vi "240312_frequency_sweep.vi"() -> ()   [LabVIEW 2015]
uses:
  <vilib>/Utility/error.llb/DialogTypeEnum.ctl
  Libraries/Stanford Research SG39x Series/Stanford Research SG39x Series.lvlib
  Libraries/SR400/SR400.lvlib
  Libraries/SRS_SR400(2013)/SRS SR400.lvlib
panel:
  out "1 cycle done":bool
  out "measure done":bool
  in  "start measurement":bool caption="Start measure"
  out "How to make setting default":string="우클릭 -> Data Operations -> Make Current Value Default"
  in  "Control":T1(tab)
  out "Parameter Explanation":string="Number of samples : 몇 번 accumulate 할 것인가에 대한 값, T SET에 해당한다.\nGate X width/delay : trigger 이후에 언제의 값을 측정할 것인가에 해당한다.\n\n>>이외에 설정값은 sub vi에서 자동으로 설정된다. 만일 바꾸고 싶다면, 해당 값을 설정하라. 세팅하면서 겪은 시행착오에 대해 sub-vi에서 건드는 값에 대해 간략히 설명해두도록 하겠다.\n>> 아래로 쭉 내용 있음\n>> 혹시라도 트리거가 제대로 들어가지 않는다면, Window->Show block diagram에서 SR400의 trigger level을 좀 낮춰보도록 하라. 거의 그럴 일은 없을 것이다.. 다만, 이 경우는 AFG를 통해 컨트롤을 한다면 참고하는 것이 좋을 것이다. \n>> Set Disc level : 이 값은 기본적으로 0.3V로 설정된다. 너무 작으면 제대로 count를 하지 못한다.\n>> Dwell time : SR400의 N_period 값이 1이 아닌 경우, 다음 스텝이 시작될 때 까지 얼마나 기다릴 것인가와 관련된다. \n                      우리의 세팅에서는 큰 의미가 없다. 한 번 trigger가 올라갔을 때 얼마나 카운팅 할 것인가에 대한 값이다.\n                      궁금하다면 바탕화면의 매뉴얼을 참고하라.\n>> N period : T_set만큼 accumulate 하는 것을 몇 번 할 것인가에 대한 값이다. 우리는 그닥 신경 안써도 된다. \n>> Gate mode : Fixed가 기본이다. 지정된 delay부터 width만큼만 값을 읽겠다는 것이다. CW는 그냥 trigger가 들어오는 시간동안 쭉 재겠다는\n                      것이다.\n>> Counter Presets : T로 되어있는데, T값을 통해 트리거하겠다는 느낌으로 생각하면 된다. 이 값은 건들 일 없을 것이다. 더 자세하게 궁금하면\n                             장비 매뉴얼을 참고하라.\n>> 나머지 값들은 장비 매뉴얼을 보거나 직접 건드려보는 편이 훨씬 더 간편하게 습득할 수 있다. \n>> EOF"
  out "String 2":string="Initialize"
  in  "SR_400_GPIB_ADDR":refnum<visa-resource-name>="GPIB0::18::INSTR"
  in  "Number of samples":dbl=5000.0
  in  "Gate B width":dbl[unit]=3e-05
  in  "Gate A width":dbl[unit]=3e-05
  in  "Gate B delay":dbl[unit]=6.03e-05
  in  "Gate A delay":dbl[unit]=3.0000000000000004e-07
  out "String":string="Measurement Setting"
  out "String 3":string="Initialize"
  in  "Final frequency (<3940MHz)":dbl=3500.0
  in  "Frequency step (MHz)":dbl=100.0
  in  "Initial frequency (<3940MHz)":dbl=2500.0 format="%#_13g"
  in  "SG394_GPIB_ADDR":refnum<visa-resource-name>="GPIB0::20::INSTR"
  in  "Modulation type":u16(ring)=7 items=["AM/ASK"=0, "FM/FSK"=1, "PM/PSK"=2, "Sweep"=3, "Pulse"=4, "Blank"=5, "QAM"=7, "CPM"=8, "VSB"=9]
  in  "N type output level value (-136dBm to 0 dBm)":dbl
  in  "start PB":bool
  in  "stop PB":bool
  in  "clock_freq (MHz)":dbl=500.0
  in  "# of Instructions":u32=4
  in  "Path to spinapi.dll":path=path "C:/SpinCore/SpinAPI/dll/spinapi64.dll"
  in  "Instructions":T2(array[cluster])=[{"Instruct Data"=0, "Op Code"=0, "Flags"=[TRUE, FALSE, FALSE, FALSE, FALSE, FALSE, FALSE, FALSE, FALSE, FALSE, FALSE, FALSE, FALSE, FALSE, FALSE, FALSE, FALSE, FALSE, FALSE, FALSE, FALSE, FALSE, FALSE, FALSE], "Comments"="", "Time (s)"=0.1}, {"Instruct Data"=0, "Op Code"=0, "Flags"=[FALSE, FALSE, FALSE, FALSE, FALSE, FALSE, FALSE, FALSE, FALSE, FALSE, FALSE, FALSE, FALSE, FALSE, FALSE, FALSE, FALSE, FALSE, FALSE, FALSE, FALSE, FALSE, FALSE, FALSE], "Comments"="", "Time (s)"=0.1}, {"Instruct Data"=0, "Op Code"=0, "Flags"=[TRUE, FALSE, FALSE, FALSE, FALSE, FALSE, FALSE, FALSE, FALSE, FALSE, FALSE, FALSE, FALSE, FALSE, FALSE, FALSE, FALSE, FALSE, FALSE, FALSE, FALSE, FALSE, FALSE, FALSE], "Comments"="", "Time (s)"=0.1}, {"Instruct Data"=0, "Op Code"=6, "Flags"=[FALSE, FALSE, FALSE, FALSE, FALSE, FALSE, FALSE, FALSE, FALSE, FALSE, FALSE, FALSE, FALSE, FALSE, FALSE, FALSE, FALSE, FALSE, FALSE, FALSE, FALSE, FALSE, FALSE, FALSE], "Comments"="", "Time (s)"=0.1}] {"Time (s)" format="%.3p"; "Op Code" items=["Continue", "Stop", "Loop", "End Loop", "JSR", "RTS", "Branch", "Long Delay", "Wait"]}
  in  "load":bool
  in  "board_num":i32
  in  "change board":bool
  out "Current frequency (MHz)":dbl
  out "Count A":i32
  out "Count B":i32
  in  "file path for measurement parameters":path=path "C:/Users/Choi group/Dropbox/Labbook/Quantum Optics/hBN/230726/attoDRY/parameters log.txt"
  in  "Parameters logging?\nMake block diagram if you want":bool=TRUE
  out "output file":refnum<file>
  in  "Measurement #":i32=11
  in  "No File Out?":bool
  in  "file folder path":path=path "C:/Users/resolution/Desktop/NV_measurements/test"
  # "1"
  # "2"
  # "3"
  # "4"
  # "5"
  # "6"
  # "7"
  # "8"
  # "9"
  # "10"
  # "11"
  # "12"
  # "13"
  # "14"
  # "15"
  # "16"
  # "17"
  # "18"
  # "19"
  # "20"
  # "21"
  # "22"
  # "23"
  # "24"
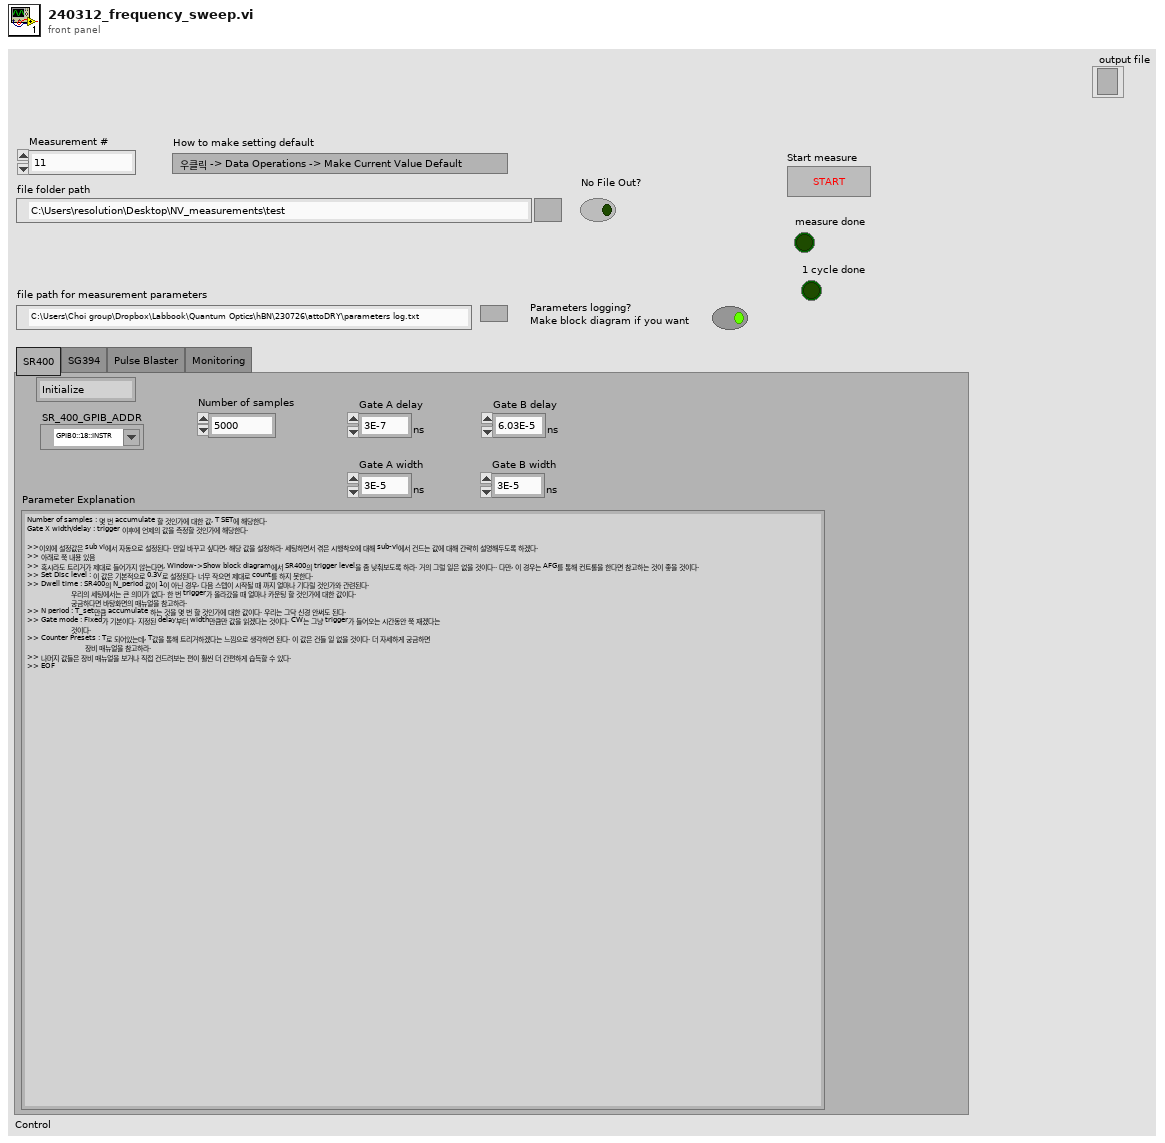
[diagram p1: front panel]
types:
  T1 = enum32{"SR400", "SG394", "Pulse Blaster", "Monitoring"}
  T2 = cluster{"Instruct Data":i32, "Op Code":i32, "Flags":bool[], "Comments":string, "Time (s)":dbl}[]
  T3 = enum16{"open", "replace", "create", "open or create", "replace or create", "replace or create with confirmation"}
  T4 = typedef "DialogTypeEnum.ctl" = enum16{"no dialog", "OK message", "continue or stop message", "auto error handling dialog", "OK message + warnings", "continue/stop + warnings"}
  T5 = enum16{"Pulse Program", "Frequency Registers", "TX Phase Registers", "RX Phase Registers"}
  T6 = cluster{"Parameter Changed from front panel":bool, "Data Ready":bool, "Scan Finished":bool, "Counter Overrun":bool, "Rate Error":bool, "Recall Error":bool, "Service Request":bool, "Command Error":bool, "Triggered":bool, "Inhibited":bool, "Counting":bool}
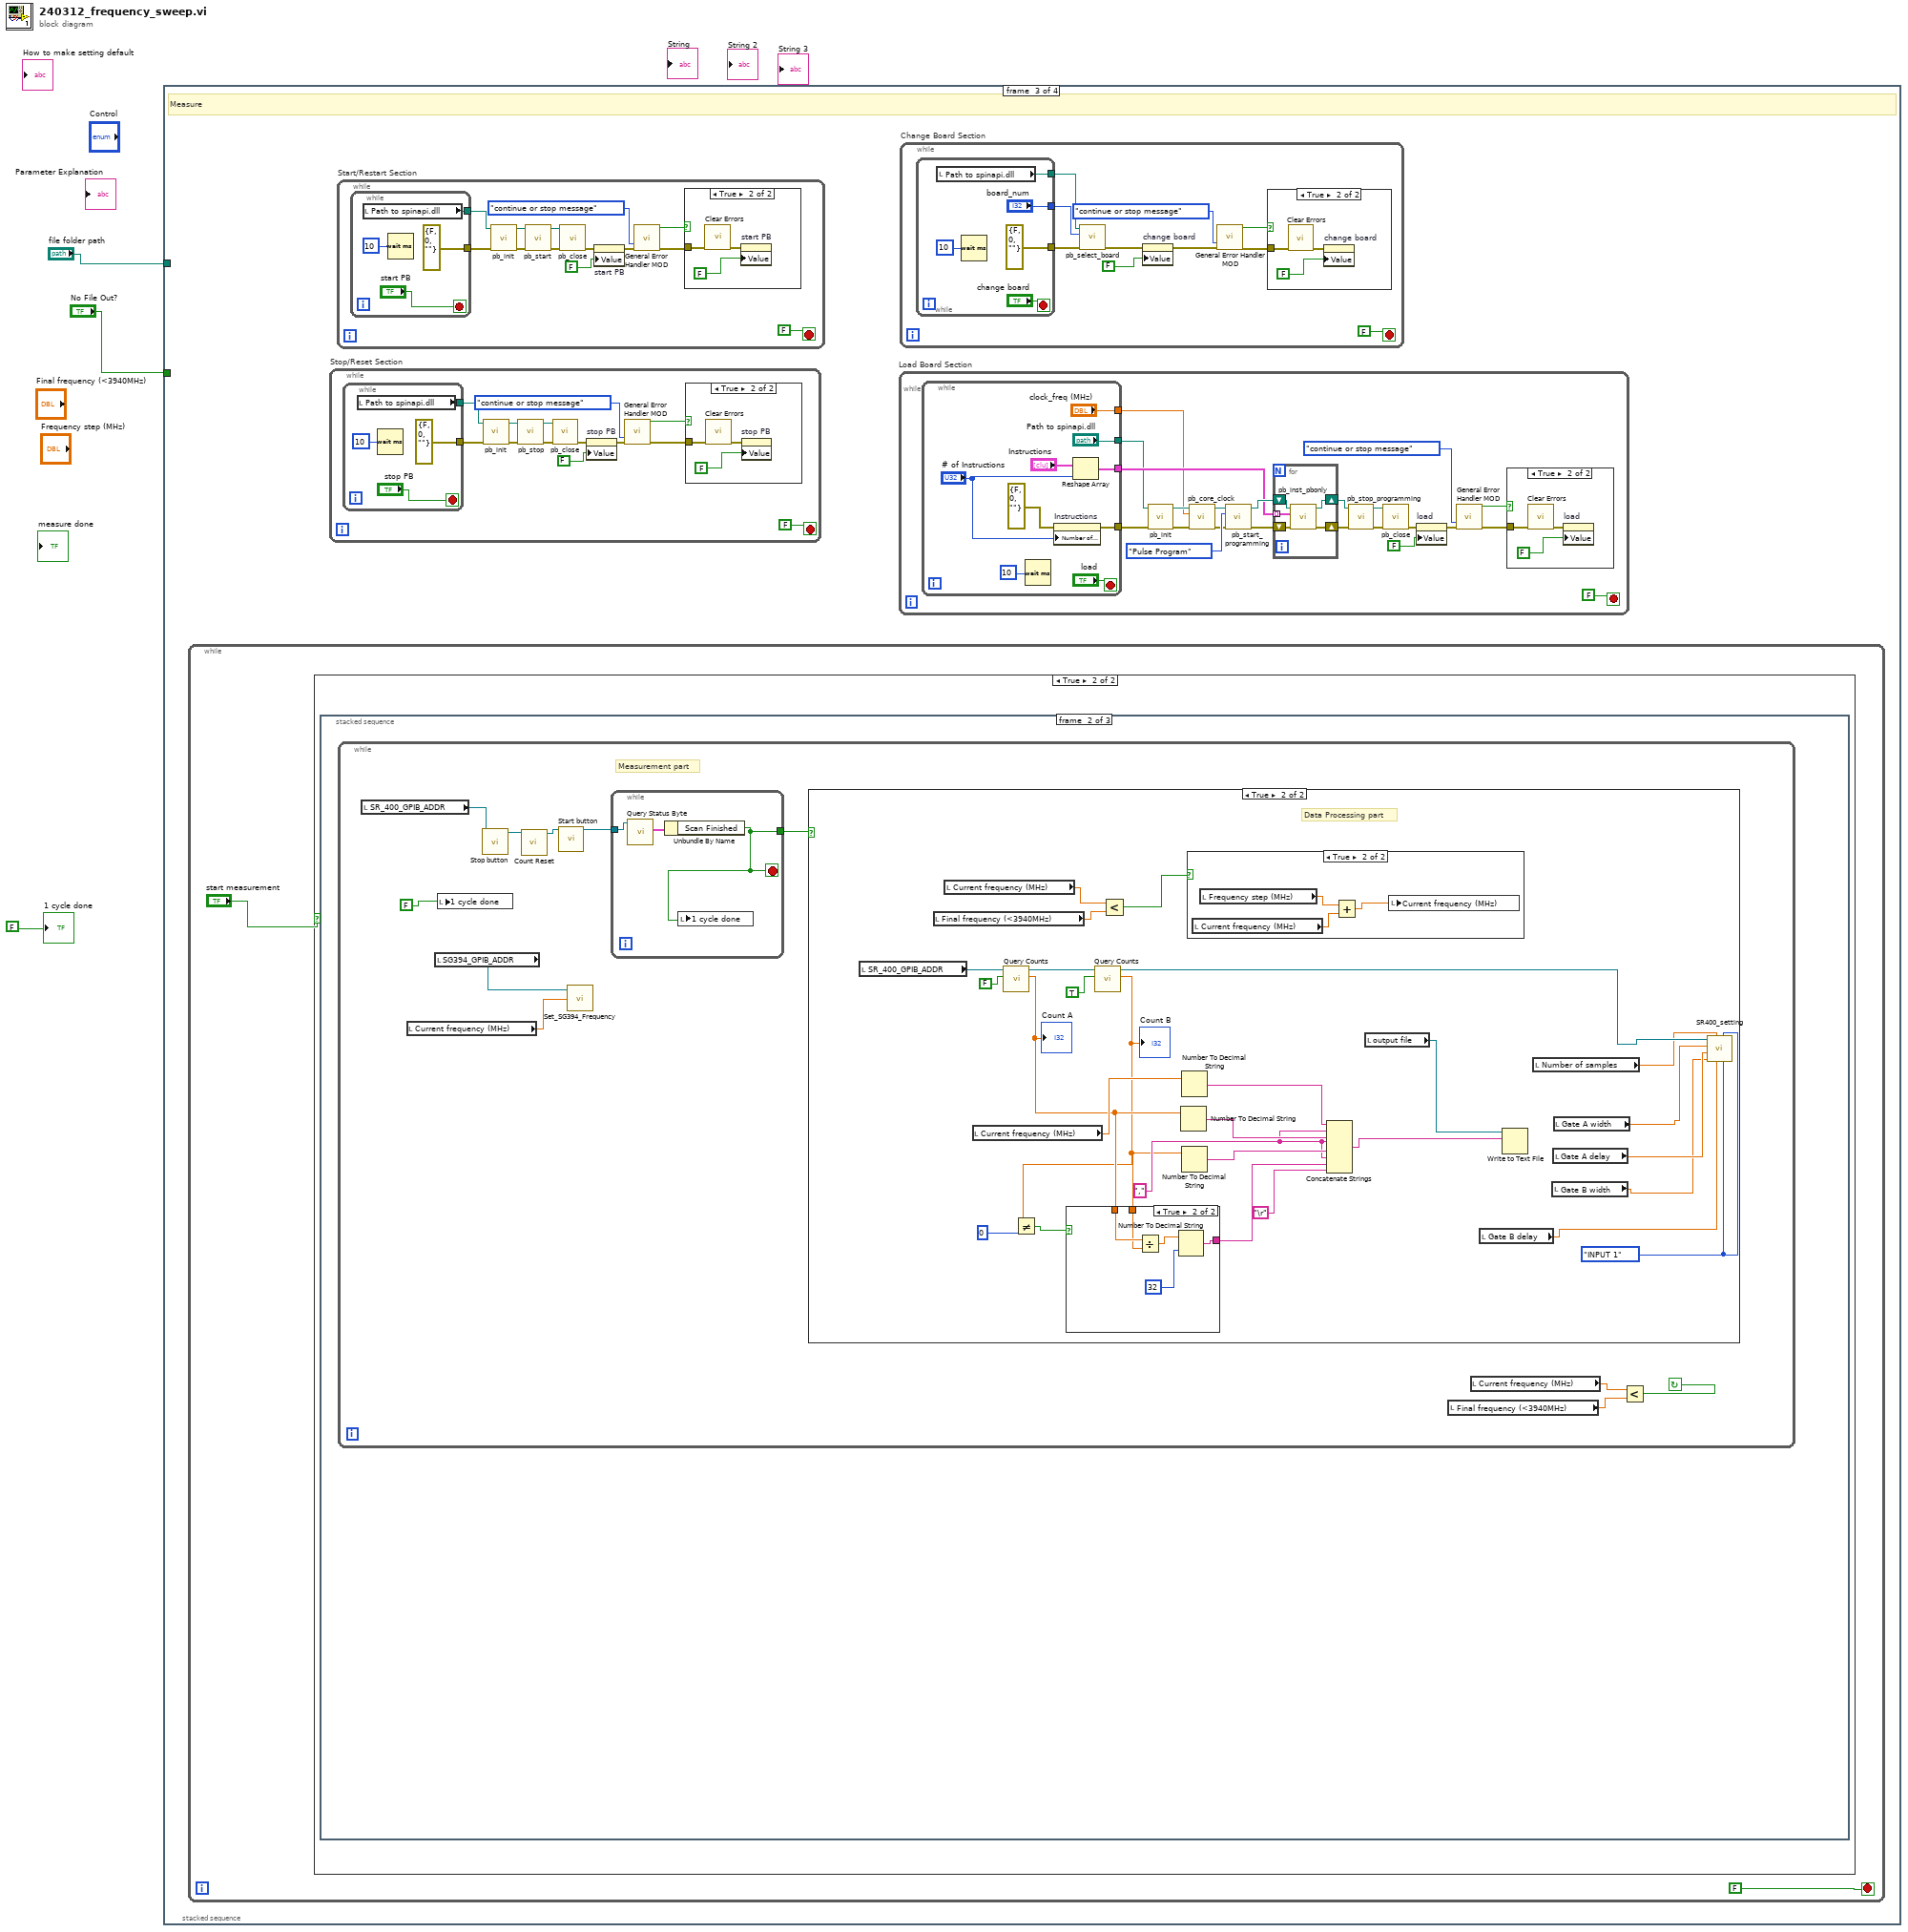
[diagram p0: block diagram]
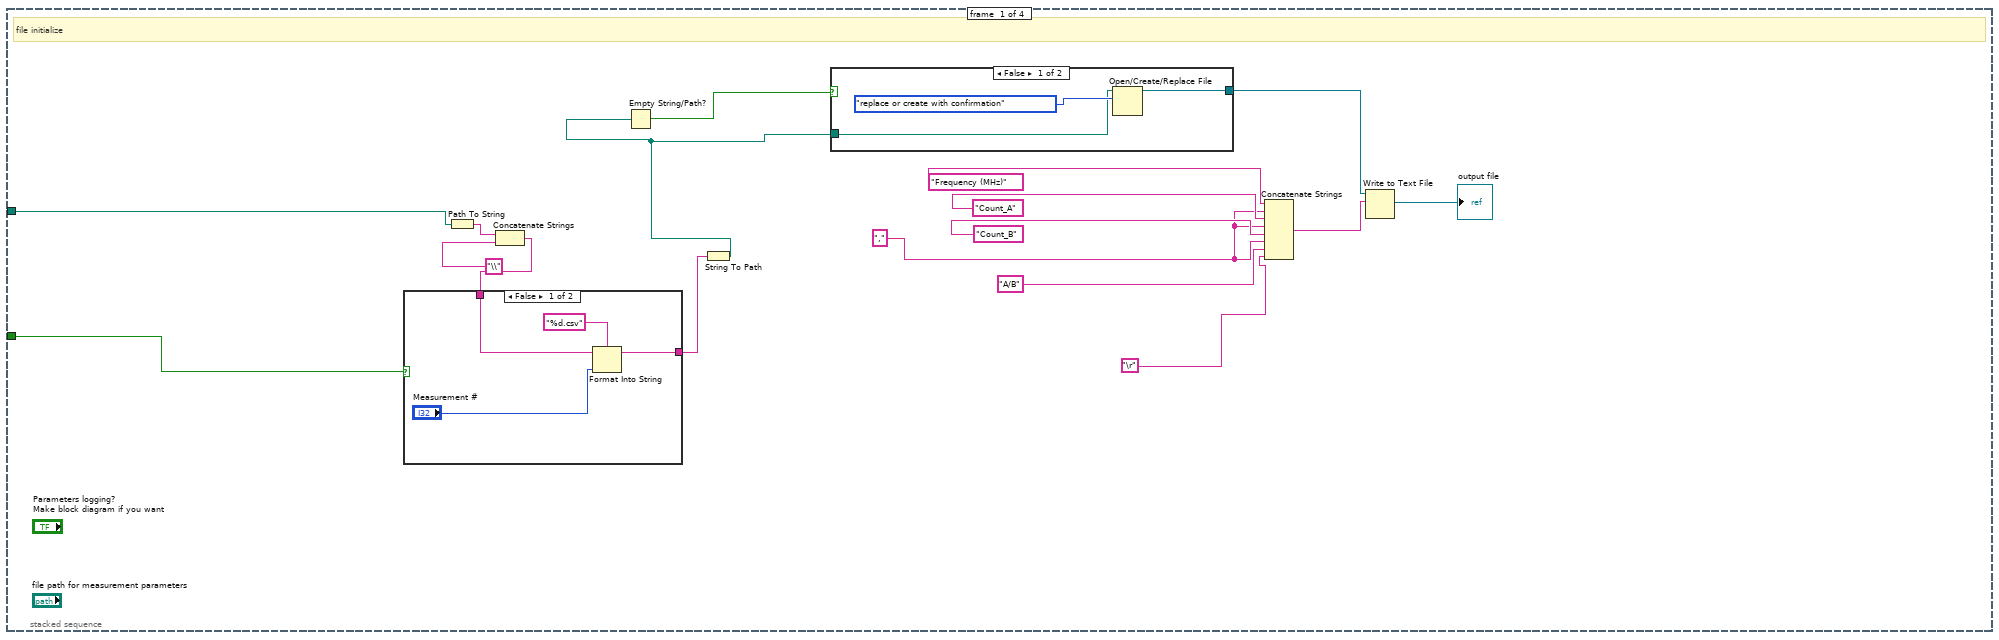
[diagram p2: hidden frame]
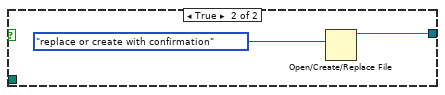
[diagram p3: hidden frame]
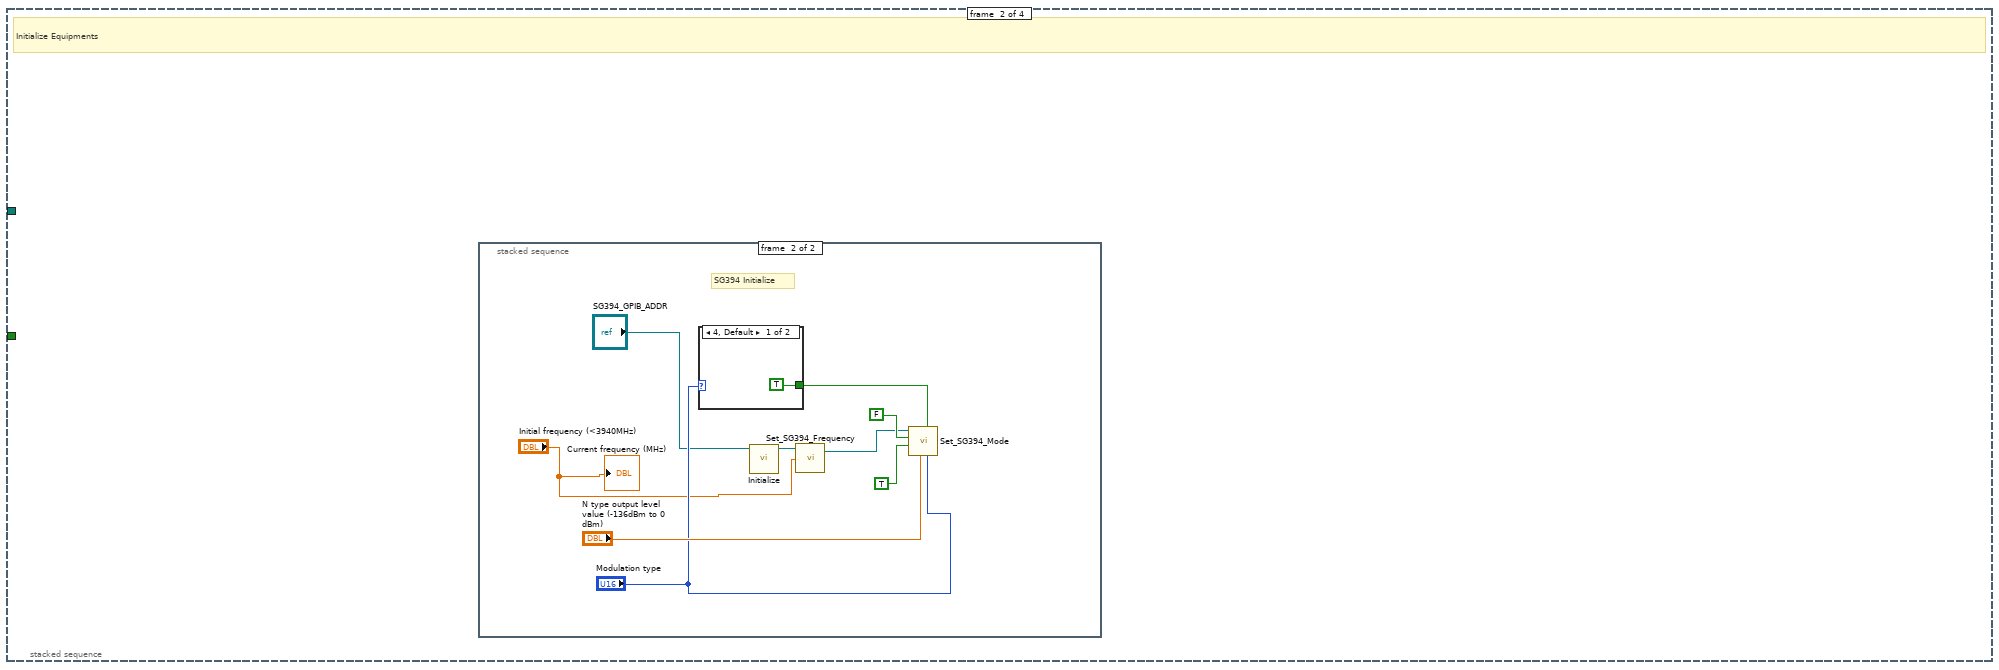
[diagram p5: hidden frame]
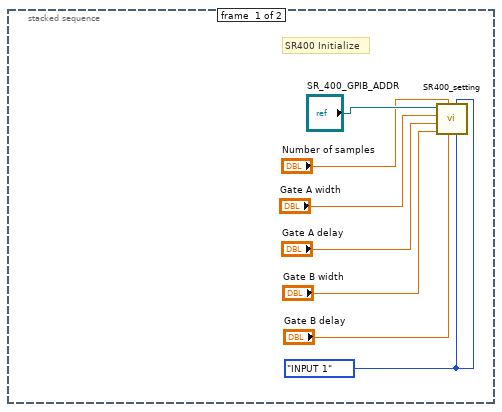
[diagram p6: hidden frame]
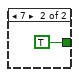
[diagram p7: hidden frame]
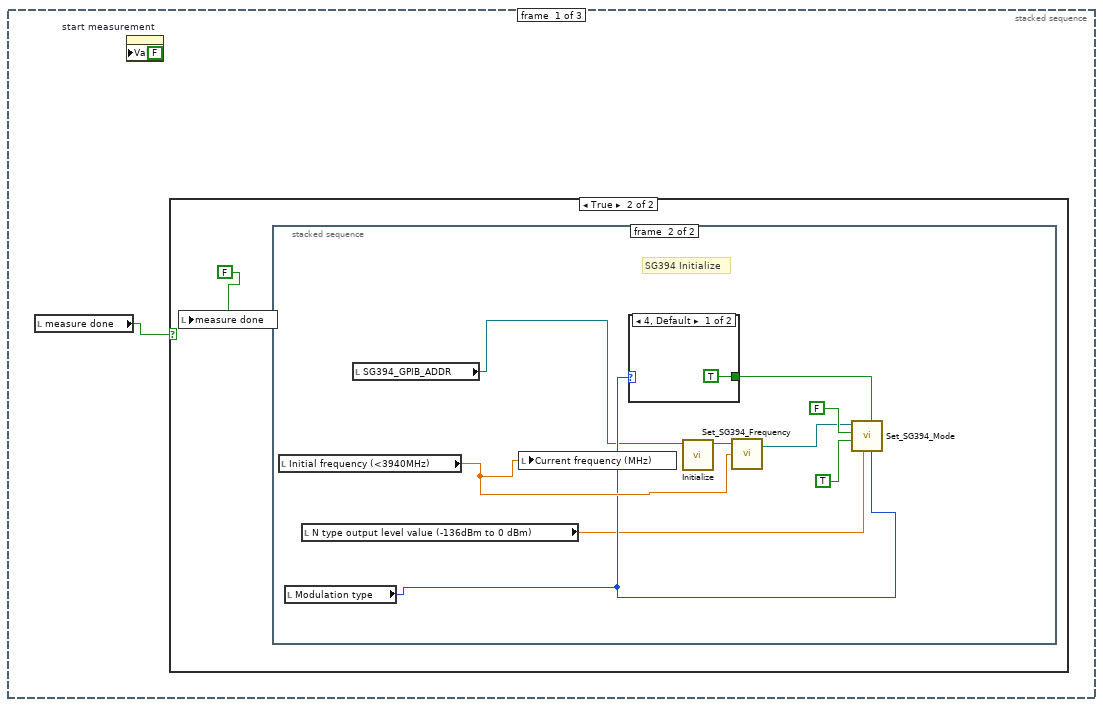
[diagram p9: hidden frame]
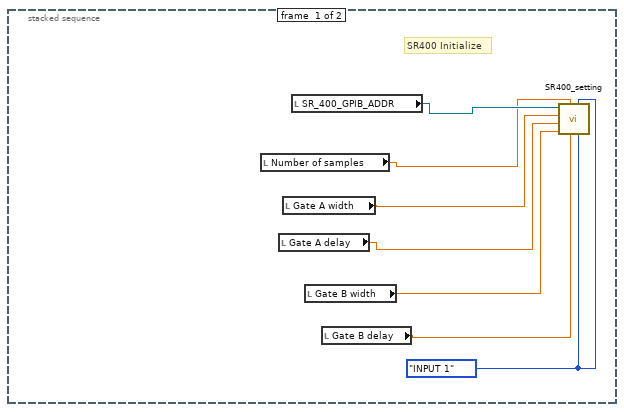
[diagram p11: hidden frame]
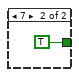
[diagram p12: hidden frame]
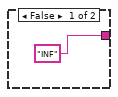
[diagram p14: hidden frame]
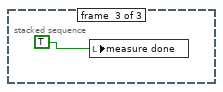
[diagram p16: hidden frame]
diagram:
  n1 = stacked-sequence {
    tunnel: "No File Out?" -> [w8 _ _ _]
    tunnel: "file folder path" -> [w7 _ _ _]
    frame #0 {
      w6 = ","
      # "file initialize"
      n2 = Path To String(path=w7) -> (string=w18:string)
      n3 = Concatenate Strings(w18, "\\" ("string")) -> (w20:string)
      n4 = case shown="False" w8 {
        tunnel: w20 -> [w27 w30]
        tunnel: [w28 w30] -> w17
        frame False {
          n5 = Format Into String(format string="%d.csv", initial string=w27, "Measurement #") -> (resulting string=w28:string)  [unwired: 1 in, 1 out]
        }
        frame True {
        }
      }
      n6 = String To Path(string=w17) -> (path=w15:path)
      n7 = Empty String/Path?(string/path=w15) -> (empty?=w16:bool)
      n8 = case shown="False" w16 {
        tunnel: [w22 w24] -> w9
        tunnel: w15 -> [w21 _]
        frame False {
          n9 = Open/Create/Replace File(file path (use dialog)=w21, operation (0:open)=T3."replace or create with confirmation") -> (refnum out=w22:refnum<file>)  [unwired: 4 in, 2 out]
        }
        frame True {
          n10 = Open/Create/Replace File(operation (0:open)=T3."replace or create with confirmation") -> (refnum out=w24:refnum<file>)  [unwired: 5 in, 2 out]
        }
      }
      n11 = Concatenate Strings("Frequency (MHz)" ("string"), w6, "Count_A" ("string"), w6, "Count_B" ("string"), w6, "A/B" ("string"), "\r") -> (w10:string)
      n12 = Write to Text File(file (use dialog)=w9, text=w10) -> (refnum out=→"output file":refnum<file>)  [unwired: 2 in, 2 out]
    }
    frame #1 {
      # "Initialize Equipments"
      n13 = stacked-sequence {
        frame #0 {
          w31 = enum16{"10 MHz", "INPUT 1", "INPUT 2", "TRIG"}."INPUT 1" ("Counter A Input")
          # "SR400 Initialize"
          n14 = call "SR400_setting.vi"("Counter B Input"=w31, "Counter A Input"=w31, "Gate B delay"="Gate B delay", "Number of samples"="Number of samples", "Gate B width"="Gate B width", "Gate A delay"="Gate A delay", "Gate A width"="Gate A width", "VISA_SR400"="SR_400_GPIB_ADDR") -> ()  [unwired: 4 in]
        }
        frame #1 {
          # "SG394 Initialize"
          n15 = case shown="4, Default" "Modulation type" {
            tunnel: [TRUE ("BNC output") TRUE ("N type output")] -> w40
            frame 4, Default {
            }
            frame 7 {
            }
          }
          n16 = call "Initialize.vi"("VISA resource name"="SG394_GPIB_ADDR") -> ("VISA resource name out"=w43:refnum<visa-resource-name>)  [unwired: 9 in, 1 out]
          n17 = call "Set_SG394_Frequency.vi"("Frequency (MHz)"="Initial frequency (<3940MHz)", "VISA resource name"=w43) -> ("VISA resource name out"=w42:refnum<visa-resource-name>)  [unwired: 1 in, 1 out]
          n18 = call "Set_SG394_Mode.vi"("Modulation type"="Modulation type", "Modulation"=w40, "N type Amplitude (-110 to 0 dBm)"="N type output level value (-136dBm to 0 dBm)", "N type output"=TRUE, "BNC output"=FALSE, "VISA resource name"=w42) -> ()  [unwired: 4 in, 2 out]
          "Current frequency (MHz)" <- "Initial frequency (<3940MHz)"
        }
      }
    }
    frame #2 {
      # "Measure"
      n19 = while {
        stop <- FALSE stop-if-true
        n20 = case shown="True" "start measurement" {
          frame False {
            # "Empty"
          }
          frame True {
            n21 = stacked-sequence {
              frame #0 {
                n22 = local read "measure done"() -> (w51:bool)
                n23 = property on="start measurement" class="Bool (strict)"("Value"=FALSE) -> ()  [unwired: 2 in, 2 out]
                n24 = case shown="True" w51 {
                  frame False {
                  }
                  frame True {
                    n25 = local write "measure done"(FALSE) -> ()
                    n26 = stacked-sequence {
                      frame #0 {
                        w60 = enum16{"10 MHz", "INPUT 1", "INPUT 2", "TRIG"}."INPUT 1" ("Counter A Input")
                        # "SR400 Initialize"
                        n27 = local read "Number of samples"() -> (w54:dbl)
                        n28 = local read "Gate A delay"() -> (w56:dbl[unit])
                        n29 = local read "Gate A width"() -> (w55:dbl[unit])
                        n30 = local read "SR_400_GPIB_ADDR"() -> (w59:refnum<visa-resource-name>)
                        n31 = local read "Gate B width"() -> (w57:dbl[unit])
                        n32 = local read "Gate B delay"() -> (w58:dbl[unit])
                        n33 = call "SR400_setting.vi"("Counter B Input"=w60, "Counter A Input"=w60, "Gate B delay"=w58, "Number of samples"=w54, "Gate B width"=w57, "Gate A delay"=w56, "Gate A width"=w55, "VISA_SR400"=w59) -> ()  [unwired: 4 in]
                      }
                      frame #1 {
                        # "SG394 Initialize"
                        n34 = local read "Initial frequency (<3940MHz)"() -> (w64:dbl)
                        n35 = local read "Modulation type"() -> (w63:u16)
                        n36 = local read "N type output level value (-136dBm to 0 dBm)"() -> (w62:dbl)
                        n37 = local read "SG394_GPIB_ADDR"() -> (w61:refnum<visa-resource-name>)
                        n38 = local write "Current frequency (MHz)"(w64) -> ()
                        n39 = case shown="4, Default" w63 {
                          tunnel: [TRUE ("BNC output") TRUE ("N type output")] -> w65
                          frame 4, Default {
                          }
                          frame 7 {
                          }
                        }
                        n40 = call "Initialize.vi"("VISA resource name"=w61) -> ("VISA resource name out"=w67:refnum<visa-resource-name>)  [unwired: 9 in, 1 out]
                        n41 = call "Set_SG394_Frequency.vi"("Frequency (MHz)"=w64, "VISA resource name"=w67) -> ("VISA resource name out"=w66:refnum<visa-resource-name>)  [unwired: 1 in, 1 out]
                        n42 = call "Set_SG394_Mode.vi"("Modulation type"=w63, "Modulation"=w65, "N type Amplitude (-110 to 0 dBm)"=w62, "N type output"=TRUE, "BNC output"=FALSE, "VISA resource name"=w66) -> ()  [unwired: 4 in, 2 out]
                      }
                    }
                  }
                }
              }
              frame #1 {
                n43 = while {
                  stop <- w76 continue-if-true
                  # "Measurement part"
                  n44 = local read "SR_400_GPIB_ADDR"() -> (w82:refnum<visa-resource-name>)
                  n45 = local read "Current frequency (MHz)"() -> (w80:dbl)
                  n46 = local read "SG394_GPIB_ADDR"() -> (w79:refnum<visa-resource-name>)
                  n47 = local write "1 cycle done"(FALSE) -> ()
                  n48 = call "Stop button.vi"("VISA resource name"=w82) -> ("VISA resource name out"=w74:refnum<visa-resource-name>)  [unwired: 9 in, 1 out]
                  n49 = call "Count Reset.vi"("VISA resource name"=w74) -> ("VISA resource name out"=w73:refnum<visa-resource-name>)  [unwired: 9 in, 1 out]
                  n50 = call "Start button.vi"("VISA resource name"=w73) -> ("VISA resource name out"=w75:refnum<visa-resource-name>)  [unwired: 9 in, 1 out]
                  n51 = call "Set_SG394_Frequency.vi"("Frequency (MHz)"=w80, "VISA resource name"=w79) -> ()  [unwired: 1 in, 2 out]
                  n52 = while {
                    tunnel: w75 -> [w120]
                    tunnel: [w119] -> w81
                    stop <- w119 stop-if-true
                    n53 = call "Query Status Byte.vi"("VISA resource name"=w120) -> ("Status Register"=w121:T6)  [unwired: 8 in, 2 out]
                    n54 = Unbundle By Name(w121) -> ("Scan Finished"=w119:bool)
                    n55 = local write "1 cycle done"(w119) -> ()
                  }
                  n56 = case shown="True" w81 {
                    frame False {
                    }
                    frame True {
                      w89 = enum16{"10 MHz", "INPUT 1", "INPUT 2", "TRIG"}."INPUT 1" ("Counter A Input")
                      w98 = ","
                      # "Data Processing part"
                      n57 = local read "SR_400_GPIB_ADDR"() -> (w90:refnum<visa-resource-name>)
                      n58 = local read "Final frequency (<3940MHz)"() -> (w109:dbl)
                      n59 = local read "Current frequency (MHz)"() -> (w108:dbl)
                      n60 = local read "Current frequency (MHz)"() -> (w103:dbl)
                      n61 = call "Query Counts.vi"("Read B?"=FALSE, "VISA resource name"=w90) -> ("Counts"=w97:dbl, "VISA resource name out"=w106:refnum<visa-resource-name>)  [unwired: 7 in, 1 out]
                      "Count A" <- w97
                      n62 = call "Query Counts.vi"("Read B?"=TRUE, "VISA resource name"=w106) -> ("Counts"=w92:dbl, "VISA resource name out"=w88:refnum<visa-resource-name>)  [unwired: 7 in, 1 out]
                      "Count B" <- w92
                      n63 = Not Equal?(x=w92, y=0) -> (x != y?=w94:bool)
                      n64 = case shown="True" w94 {
                        tunnel: w92 -> [_ w111]
                        tunnel: w97 -> [_ w112]
                        tunnel: ["INF" w113] -> w91
                        frame False {
                        }
                        frame True {
                          n65 = Divide(x=w112, y=w111) -> (x/y=w115:dbl)
                          n66 = Number To Decimal String(number=w115, width (-)=32) -> (decimal integer string=w113:string)
                        }
                      }
                      n67 = Less?(x=w108, y=w109) -> (x < y?=w107:bool)
                      n68 = Number To Decimal String(number=w97) -> (decimal integer string=w101:string)  [unwired: 1 in]
                      n69 = Number To Decimal String(number=w103) -> (decimal integer string=w102:string)  [unwired: 1 in]
                      n70 = Number To Decimal String(number=w92) -> (decimal integer string=w100:string)  [unwired: 1 in]
                      n71 = case shown="True" w107 {
                        frame False {
                        }
                        frame True {
                          n72 = local read "Current frequency (MHz)"() -> (w117:dbl)
                          n73 = local read "Frequency step (MHz)"() -> (w118:dbl)
                          n74 = Add(x=w118, y=w117) -> (x+y=w116:dbl)
                          n75 = local write "Current frequency (MHz)"(w116) -> ()
                        }
                      }
                      n76 = Concatenate Strings(w102, w98, w101, w98, w100, w98, w91, "\r") -> (w96:string)
                      n77 = local read "output file"() -> (w95:refnum<file>)
                      n78 = local read "Gate B delay"() -> (w83:dbl[unit])
                      n79 = Write to Text File(file (use dialog)=w95, text=w96) -> ()  [unwired: 2 in, 3 out]
                      n80 = local read "Number of samples"() -> (w87:dbl)
                      n81 = local read "Gate B width"() -> (w84:dbl[unit])
                      n82 = local read "Gate A delay"() -> (w86:dbl[unit])
                      n83 = local read "Gate A width"() -> (w85:dbl[unit])
                      n84 = call "SR400_setting.vi"("Counter B Input"=w89, "Counter A Input"=w89, "Gate B delay"=w83, "Number of samples"=w87, "Gate B width"=w84, "Gate A delay"=w86, "Gate A width"=w85, "VISA_SR400"=w88) -> ()  [unwired: 4 in]
                    }
                  }
                  n85 = local read "Final frequency (<3940MHz)"() -> (w77:dbl)
                  n86 = local read "Current frequency (MHz)"() -> (w78:dbl)
                  n87 = Less?(x=w78, y=w77) -> (x < y?=w76:bool)
                }
              }
              frame #2 {
                n88 = local write "measure done"(TRUE) -> ()
              }
            }
          }
        }
      }
      n89 = while "Stop/Reset Section" {
        stop <- FALSE stop-if-true
        n90 = while {
          tunnel: [errorcluster {"status"=FALSE, "code"=0, "source"=""} ("error in (no error)")] -> w171
          tunnel: [w179] -> w162
          stop <- "stop PB" stop-if-true
          n91 = local read "Path to spinapi.dll"() -> (w179:path)
          n92 = Wait (ms)(milliseconds to wait=u32 10) -> ()  [unwired: 1 out]
        }
        n93 = call "pb_init.vi"("error in (no error)"=w171, "path in"=w162) -> ("error out"=w170:errorcluster, "path out"=w173:path)  [unwired: 1 in, 7 out]
        n94 = call "pb_stop.vi"("error in (no error)"=w170, "path in"=w173) -> ("error out"=w169:errorcluster, "path out"=w174:path)  [unwired: 8 out]
        n95 = call "pb_close.vi"("error in (no error)"=w169, "path in"=w174) -> ("error out"=w168:errorcluster)  [unwired: 9 out]
        n96 = property on="stop PB" class="Bool (strict)"(error in=w168, "Value"=FALSE ("stop")) -> (error out=w167:errorcluster)  [unwired: 1 in, 1 out]
        n97 = call "General Error Handler MOD.vi"("type of dialog (OK msg:1)"=DialogTypeEnum."continue or stop message", "error in (no error)"=w167) -> ("STOP?"=w164:bool, "error out"=w163:errorcluster)  [unwired: 12 out]
        n98 = case shown="True" w164 {
          tunnel: w163 -> [_ w177]
          frame False {
          }
          frame True {
            n99 = call <vilib>:"Clear Errors.vi"("error in (no error)"=w177) -> ("error out"=w175:errorcluster)  [unwired: 1 in, 5 out]
            n100 = property on="stop PB" class="Bool (strict)"(error in=w175, "Value"=FALSE ("Waiting for Data Acquisition")) -> ()  [unwired: 1 in, 2 out]
          }
        }
      }
      n101 = while "Start/Restart Section" {
        stop <- FALSE stop-if-true
        n102 = while {
          tunnel: [errorcluster {"status"=FALSE, "code"=0, "source"=""} ("error in (no error)")] -> w209
          tunnel: [w217] -> w200
          stop <- "start PB" stop-if-true
          n103 = local read "Path to spinapi.dll"() -> (w217:path)
          n104 = Wait (ms)(milliseconds to wait=u32 10) -> ()  [unwired: 1 out]
        }
        n105 = call "pb_init.vi"("error in (no error)"=w209, "path in"=w200) -> ("error out"=w208:errorcluster, "path out"=w211:path)  [unwired: 1 in, 7 out]
        n106 = call "pb_start.vi"("error in (no error)"=w208, "path in"=w211) -> ("error out"=w207:errorcluster, "path out"=w212:path)  [unwired: 1 in, 7 out]
        n107 = call "pb_close.vi"("error in (no error)"=w207, "path in"=w212) -> ("error out"=w206:errorcluster)  [unwired: 9 out]
        n108 = property on="start PB" class="Bool (strict)"(error in=w206, "Value"=FALSE ("start/restart")) -> (error out=w205:errorcluster)  [unwired: 1 in, 1 out]
        n109 = call "General Error Handler MOD.vi"("type of dialog (OK msg:1)"=DialogTypeEnum."continue or stop message", "error in (no error)"=w205) -> ("STOP?"=w202:bool, "error out"=w201:errorcluster)  [unwired: 12 out]
        n110 = case shown="True" w202 {
          tunnel: w201 -> [_ w215]
          frame False {
          }
          frame True {
            n111 = call <vilib>:"Clear Errors.vi"("error in (no error)"=w215) -> ("error out"=w213:errorcluster)  [unwired: 1 in, 5 out]
            n112 = property on="start PB" class="Bool (strict)"(error in=w213, "Value"=FALSE ("Waiting for Data Acquisition")) -> ()  [unwired: 1 in, 2 out]
          }
        }
      }
      n113 = while "Load Board Section" {
        stop <- FALSE stop-if-true
        n114 = while {
          tunnel: [w156] -> w139
          tunnel: [w157] -> w141
          tunnel: ["Path to spinapi.dll"] -> w124
          tunnel: ["clock_freq (MHz)"] -> w123
          stop <- "load" stop-if-true
          n115 = Wait (ms)(milliseconds to wait=u32 10) -> ()  [unwired: 1 out]
          n116 = property on="Instructions" class="Arr (strict)"(error in=errorcluster {"status"=FALSE, "code"=0, "source"=""} ("error in (no error)"), "Number of Columns"="# of Instructions") -> (error out=w156:errorcluster)  [unwired: 1 in, 1 out]
          n117 = Reshape Array("Instructions", "# of Instructions") -> (w157:T2)
        }
        n118 = call "pb_init.vi"("error in (no error)"=w139, "path in"=w124) -> ("error out"=w126:errorcluster, "path out"=w128:path)  [unwired: 2 in, 6 out]
        n119 = call "pb_core_clock.vi"("error in (no error)"=w126, "clock_freq (MHz)"=w123, "path in"=w128) -> ("error out"=w125:errorcluster, "path out"=w127:path)  [unwired: 7 in]
        n120 = call "pb_start_programming.vi"("error in (no error)"=w125, "Device"=T5."Pulse Program", "path in"=w127) -> ("error out"=w137:errorcluster, "path out"=w144:path)  [unwired: 1 in, 6 out]
        n121 = for {
          tunnel: w141 -> [w149] mode=indexing
          shift-right: [w151] -> w140
          shift-left: w144 -> [w152]
          shift-right: [w148] -> w136
          shift-left: w137 -> [w150]
          n122 = call "pb_inst_pbonly.vi"("error in (no error)"=w150, "PB Instruction"=w149, "path in"=w152) -> ("error out"=w148:errorcluster, "path out"=w151:path)  [unwired: 2 in, 5 out]
        }
        n123 = call "pb_stop_programming.vi"("error in (no error)"=w136, "path in"=w140) -> ("error out"=w135:errorcluster, "path out"=w143:path)  [unwired: 1 in, 7 out]
        n124 = call "pb_close.vi"("error in (no error)"=w135, "path in"=w143) -> ("error out"=w133:errorcluster)  [unwired: 9 out]
        n125 = property on="load" class="Bool (strict)"(error in=w133, "Value"=FALSE ("load")) -> (error out=w132:errorcluster)  [unwired: 1 in, 1 out]
        n126 = call "General Error Handler MOD.vi"("type of dialog (OK msg:1)"=DialogTypeEnum."continue or stop message", "error in (no error)"=w132) -> ("STOP?"=w129:bool, "error out"=w130:errorcluster)  [unwired: 12 out]
        n127 = case shown="True" w129 {
          tunnel: w130 -> [_ w147]
          frame False {
          }
          frame True {
            n128 = call <vilib>:"Clear Errors.vi"("error in (no error)"=w147) -> ("error out"=w145:errorcluster)  [unwired: 1 in, 5 out]
            n129 = property on="load" class="Bool (strict)"(error in=w145, "Value"=FALSE ("Waiting for Data Acquisition")) -> ()  [unwired: 1 in, 2 out]
          }
        }
      }
      n130 = while "Change Board Section" {
        stop <- FALSE stop-if-true
        n131 = while {
          tunnel: [errorcluster {"status"=FALSE, "code"=0, "source"=""} ("error in (no error)")] -> w191
          tunnel: ["board_num"] -> w190
          tunnel: [w195] -> w182
          stop <- "change board" stop-if-true
          n132 = local read "Path to spinapi.dll"() -> (w195:path)
          n133 = Wait (ms)(milliseconds to wait=u32 10) -> ()  [unwired: 1 out]
        }
        n134 = call "pb_select_board.vi"("error in (no error)"=w191, "board_num"=w190, "path in"=w182) -> ("error out"=w188:errorcluster)  [unwired: 8 out]
        n135 = property on="change board" class="Bool (strict)"(error in=w188, "Value"=FALSE ("change board")) -> (error out=w187:errorcluster)  [unwired: 1 in, 1 out]
        n136 = call "General Error Handler MOD.vi"("type of dialog (OK msg:1)"=DialogTypeEnum."continue or stop message", "error in (no error)"=w187) -> ("STOP?"=w184:bool, "error out"=w183:errorcluster)  [unwired: 12 out]
        n137 = case shown="True" w184 {
          tunnel: w183 -> [_ w194]
          frame False {
          }
          frame True {
            n138 = call <vilib>:"Clear Errors.vi"("error in (no error)"=w194) -> ("error out"=w192:errorcluster)  [unwired: 1 in, 5 out]
            n139 = property on="change board" class="Bool (strict)"(error in=w192, "Value"=FALSE ("Waiting for Data Acquisition")) -> ()  [unwired: 1 in, 2 out]
          }
        }
      }
    }
    frame #3 {
      # "close file"
      n140 = local read "output file"() -> (w220:refnum<file>)
      n141 = Close File(refnum=w220) -> ()  [unwired: 1 in, 2 out]
    }
  }
  "1 cycle done" <- FALSE
